vi "Multiplex to number.vi"(11 "Start-Stop4 Multyplex":T1) -> (3 "Numeric":u32)   [LabVIEW 2012]
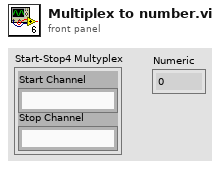
[diagram p1: front panel]
types:
  T1 = cluster{"Start Channel":string, "Stop Channel":string}
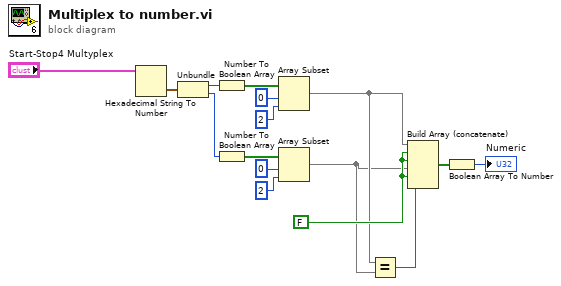
[diagram p0: block diagram]
diagram:
  w14 = FALSE
  n1 = Hexadecimal String To Number(string="Start-Stop4 Multyplex") -> (number=w11:cluster{"Start Channel":u32, "Stop Channel":u32})  [unwired: 2 in, 1 out]
  n2 = Unbundle(w11) -> ("Start Channel"=w12:u32, "Stop Channel"=w13:u32)
  n3 = Number To Boolean Array(number=w12) -> (Boolean array=w5:bool[])
  n4 = Number To Boolean Array(number=w13) -> (Boolean array=w4:bool[])
  n5 = Array Subset(array=w5, index=0, length=2) -> (w3:bool[])
  n6 = Array Subset(array=w4, index=0, length=2) -> (w2:bool[])
  n7 = Equal?(x=w3, y=w2) -> (x = y?=w1:bool)
  n8 = Build Array (concatenate)(w3, w14, w14, w2, w14, w1) -> (w15:bool[])
  n9 = Boolean Array To Number(Boolean array=w15) -> (number=→"Numeric":u32)
